vi "Log Data U16.vi"(0 "TDMS Log In":refnum<class "TDMS Logger.lvclass">, 5 "Group Name":string, 7 "Channels Names":string[](array[string]), 9 "U16 Data":u16[][](array[numeric]), 11 "Error In":errorcluster) -> (4 "TDMS Log Out":refnum<class "TDMS Logger.lvclass">, 15 "Error Out":errorcluster)   [LabVIEW 2019, in "TDMS Logger.lvlib" / "TDMS Logger.lvclass"]
doc: "Send U16 data to asynch logger."
uses:
  TDMS Logger.lvclass
  TDMS Logger.lvclass/TDMS Logger.ctl
  _Typedefs/Data Type.ctl
  _Typedefs/Log Message.ctl
  _Typedefs/Log Action.ctl
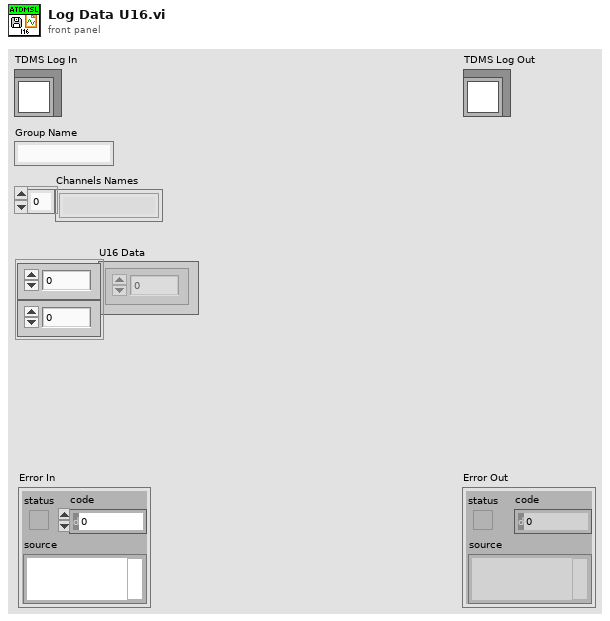
[diagram p1: front panel]
types:
  T1 = typedef "TDMS Logger.lvlib/TDMS Logger.lvclass/Data Type.ctl" = enum16{"I16", "I8", "String", "U16", "U8", "Waveform", "Double", "Single"}
  T2 = typedef "TDMS Logger.lvlib/TDMS Logger.lvclass/Log Message.ctl" = cluster{"Log Action":T3, "Variant":variant, "Data Type":T1, "Group Name":string, "Channels Names":string[]}
  T3 = typedef "TDMS Logger.lvlib/TDMS Logger.lvclass/Log Action.ctl" = enum16{"Handle Old Files", "Status Update", "Stop", "Log Data", "Initialize"}
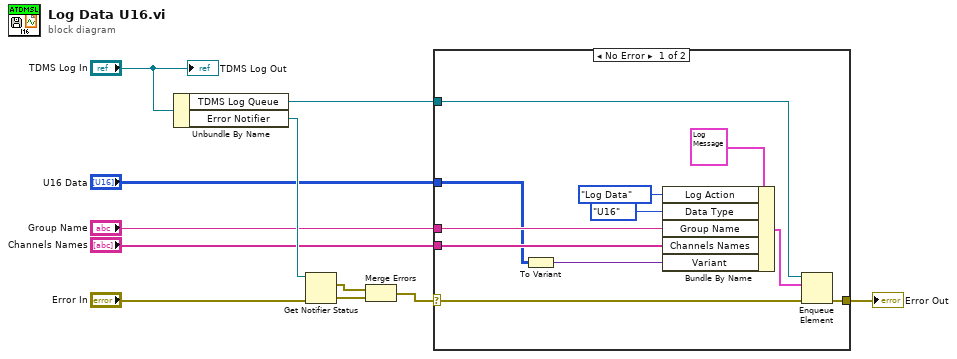
[diagram p0: block diagram]
diagram:
  n1 = Unbundle By Name("TDMS Log In") -> ("TDMS Log Queue"=w10:refnum<queue>, "Error Notifier"=w7:refnum<notifier>)
  n2 = Get Notifier Status(notifier=w7, error in (no error)="Error In") -> (current notification=w4:errorcluster, error out=w5:errorcluster)  [unwired: 3 out]
  n3 = Merge Errors(w4, w5) -> (w6:errorcluster)
  n4 = case shown="No Error" w6 {
    selector: w6 -> [w16 w23]
    tunnel: [w14 w23] -> w11
    tunnel: w10 -> [w15 _]
    tunnel: "U16 Data" -> [w12 _]
    tunnel: "Group Name" -> [w18 _]
    tunnel: "Channels Names" -> [w17 _]
    frame No Error {
      n5 = To Variant(anything=w12) -> (Variant=w13:variant)
      n6 = Bundle By Name(cluster=T2 {"Log Action"=enum."Stop", "Variant"=variant, "Data Type"=enum."String", "Group Name"="", "Channels Names"=[]} ("element"), "Log Action"=Log_Action."Log Data", "Data Type"=Data_Type."U16", "Group Name"=w18, "Channels Names"=w17, "Variant"=w13) -> (w21:T2)
      n7 = Enqueue Element(queue=w15, element=w21, error in (no error)=w16) -> (error out=w14:errorcluster)  [unwired: 1 in, 2 out]
    }
    frame Error {
    }
  }
  "Error Out" <- w11
  "TDMS Log Out" <- "TDMS Log In"
